vi "Initial.vi"() -> (0 "error out":errorcluster, 1 "DevAlloc":i32, 2 "DeviceID":u32, 3 "path out":path, 4 "SerialNumber":i32, 5 "DMD Type":string, 7 "DeviceIdPtr":u32)   [LabVIEW 2016]
panel:
  # "This subvi automatically detects the DMD connected to the host.\nThe DMD type, Device ID, DevAlloc, and Serial Number are returned."
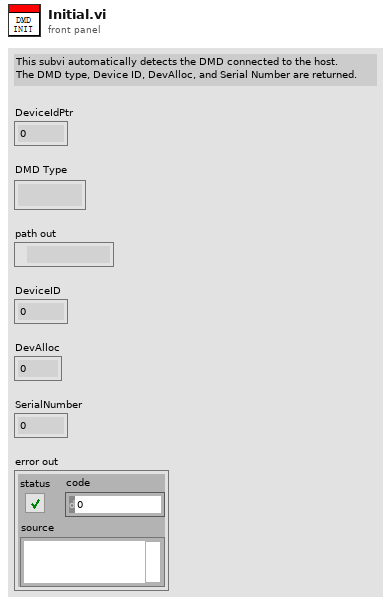
[diagram p1: front panel]
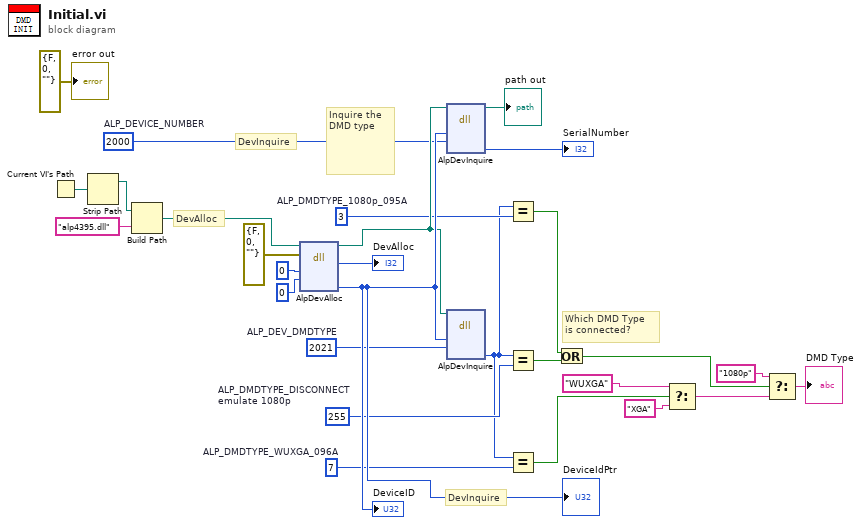
[diagram p0: block diagram]
diagram:
  w12 = u32 7  # ALP_DMDTYPE_WUXGA_096A
  w8 = u32 255  # ALP_DMDTYPE_DISCONNECT emulate 1080p
  w9 = u32 3  # ALP_DMDTYPE_1080p_095A
  w7 = 2021  # ALP_DEV_DMDTYPE
  w5 = 2000  # ALP_DEVICE_NUMBER
  # "Which DMD Type\nis connected?"
  # "DevInquire"
  # "Inquire the DMD type"
  # "DevInquire"
  # "DevAlloc"
  n1 = Current VI's Path() -> (path=w19:path)
  n2 = Strip Path(path=w19) -> (stripped path=w21:path)  [unwired: 1 out]
  n3 = Build Path(base path=w21, name or relative path="alp4395.dll") -> (appended path=w22:path)
  n4 = dll-call lib="?" fn="AlpDevAlloc"(path in=w22, error in=errorcluster {"status"=FALSE, "code"=0, "source"=""} ("error in (no error)"), "DeviceNum"=0, "InitFlag"=0) -> (path out=w16:path, "return type"=→"DevAlloc":i32, "DeviceIdPtr"=w18:u32)  [unwired: 4 in, 1 out]
  "DeviceID" <- w18
  "DeviceIdPtr" <- w18
  n5 = dll-call lib="?" fn="AlpDevInquire"(path in=w16, "DeviceId"=w18, "InquireType"=w5) -> (path out=→"path out":path, "UserVar"=→"SerialNumber":i32)  [unwired: 6 in, 1 out]
  n6 = dll-call lib="?" fn="AlpDevInquire"(path in=w16, "DeviceId"=w18, "InquireType"=w7) -> ("UserVar"=w1:i32)  [unwired: 6 in, 2 out]
  n7 = Equal?(x=w1, y=w9) -> (x = y?=w10:bool)
  n8 = Equal?(x=w1, y=w8) -> (x = y?=w11:bool)
  n9 = Equal?(x=w1, y=w12) -> (x = y?=w13:bool)
  n10 = Or(x=w10, y=w11) -> (x .or. y?=w24:bool)
  n11 = Select(t="WUXGA", s=w13, f="XGA") -> (s? t:f=w26:string)
  n12 = Select(t="1080p", s=w24, f=w26) -> (s? t:f=→"DMD Type":string)
  "error out" <- errorcluster {"status"=FALSE, "code"=0, "source"=""} ("error out")
